vi "2D plot_take linecut_average.vi"() -> ()   [LabVIEW 2016]
uses:
  <vilib>/Analysis/baseanly.llb/Mean (DBL).vi
  <vilib>/Analysis/NI_AALPro.lvlib
  <vilib>/Analysis/NI_AALBase.lvlib
  <vilib>/gmath/NI_Gmath.lvlib
  <userlib>/_OpenG.lib/array/array.llb/Delete Elements from 1D Array (DBL)__ogtk.vi
  <userlib>/_OpenG.lib/array/array.llb/Search 1D Array (DBL)__ogtk.vi
  <vilib>/Analysis/NI_AAL_SigProc.lvlib
panel:
  in  "threshold 2":dbl format="%0.2f"
  in  "width 2":i32=3 min=3
  out "trandconductance 2":cluster{dbl[], dbl[]}[](graph)
  out "Indices of Elements 2":i32[](array[numeric])
  out "Array 3":dbl[](array[numeric])
  out "array w/ subset deleted 2":dbl[](array[numeric]) format="%.2f"
  out "resampled G 3":cluster{dbl[], dbl[]}(graph)
  out "trandconductance":cluster{dbl[], dbl[]}[](graph)
  out "Array":i32[](array[numeric])
  in  "Tab Control":enum32{"Page 1", "Page 2"}(tab)
  in  "Input transconductance":dbl[][](graph)
  in  "Number of cursors":i32[](array[numeric])=[0, 1, 2, 3]
  in  "input cond":dbl[][](graph)
  out "XY Graph":cluster{"xi used":dbl[], "yi":dbl[]}[](graph)
  out "Trans intensity":dbl[][](graph)
  out "G":cluster{dbl[], dbl[]}[](graph)
  out "Cond intensity":dbl[][](graph)
  in  "alpha":dbl=1.0 format="%#_13g"
  out "mean G change":dbl=3.541411002779411 format="%0.2f"
  out "old average G":cluster{dbl[], dbl[]}[](graph)
  out "delta y1":dbl format="%#_6p"
  out "delta y2":dbl format="%#_6p"
  out "resampled G":cluster{dbl[], dbl[]}[](graph)
  out "resampled average G":cluster{dbl[], dbl[]}[](graph)
  in  "max value":dbl
  in  "min value":dbl
  in  "X Step":dbl=0.00025 format="%#_13g"
  in  "pad array T\ninterpolate F":bool
  out "shifted + avg":cluster{dbl[], dbl[]}[](graph)
  # "29.2    .139\n60.4    .129"
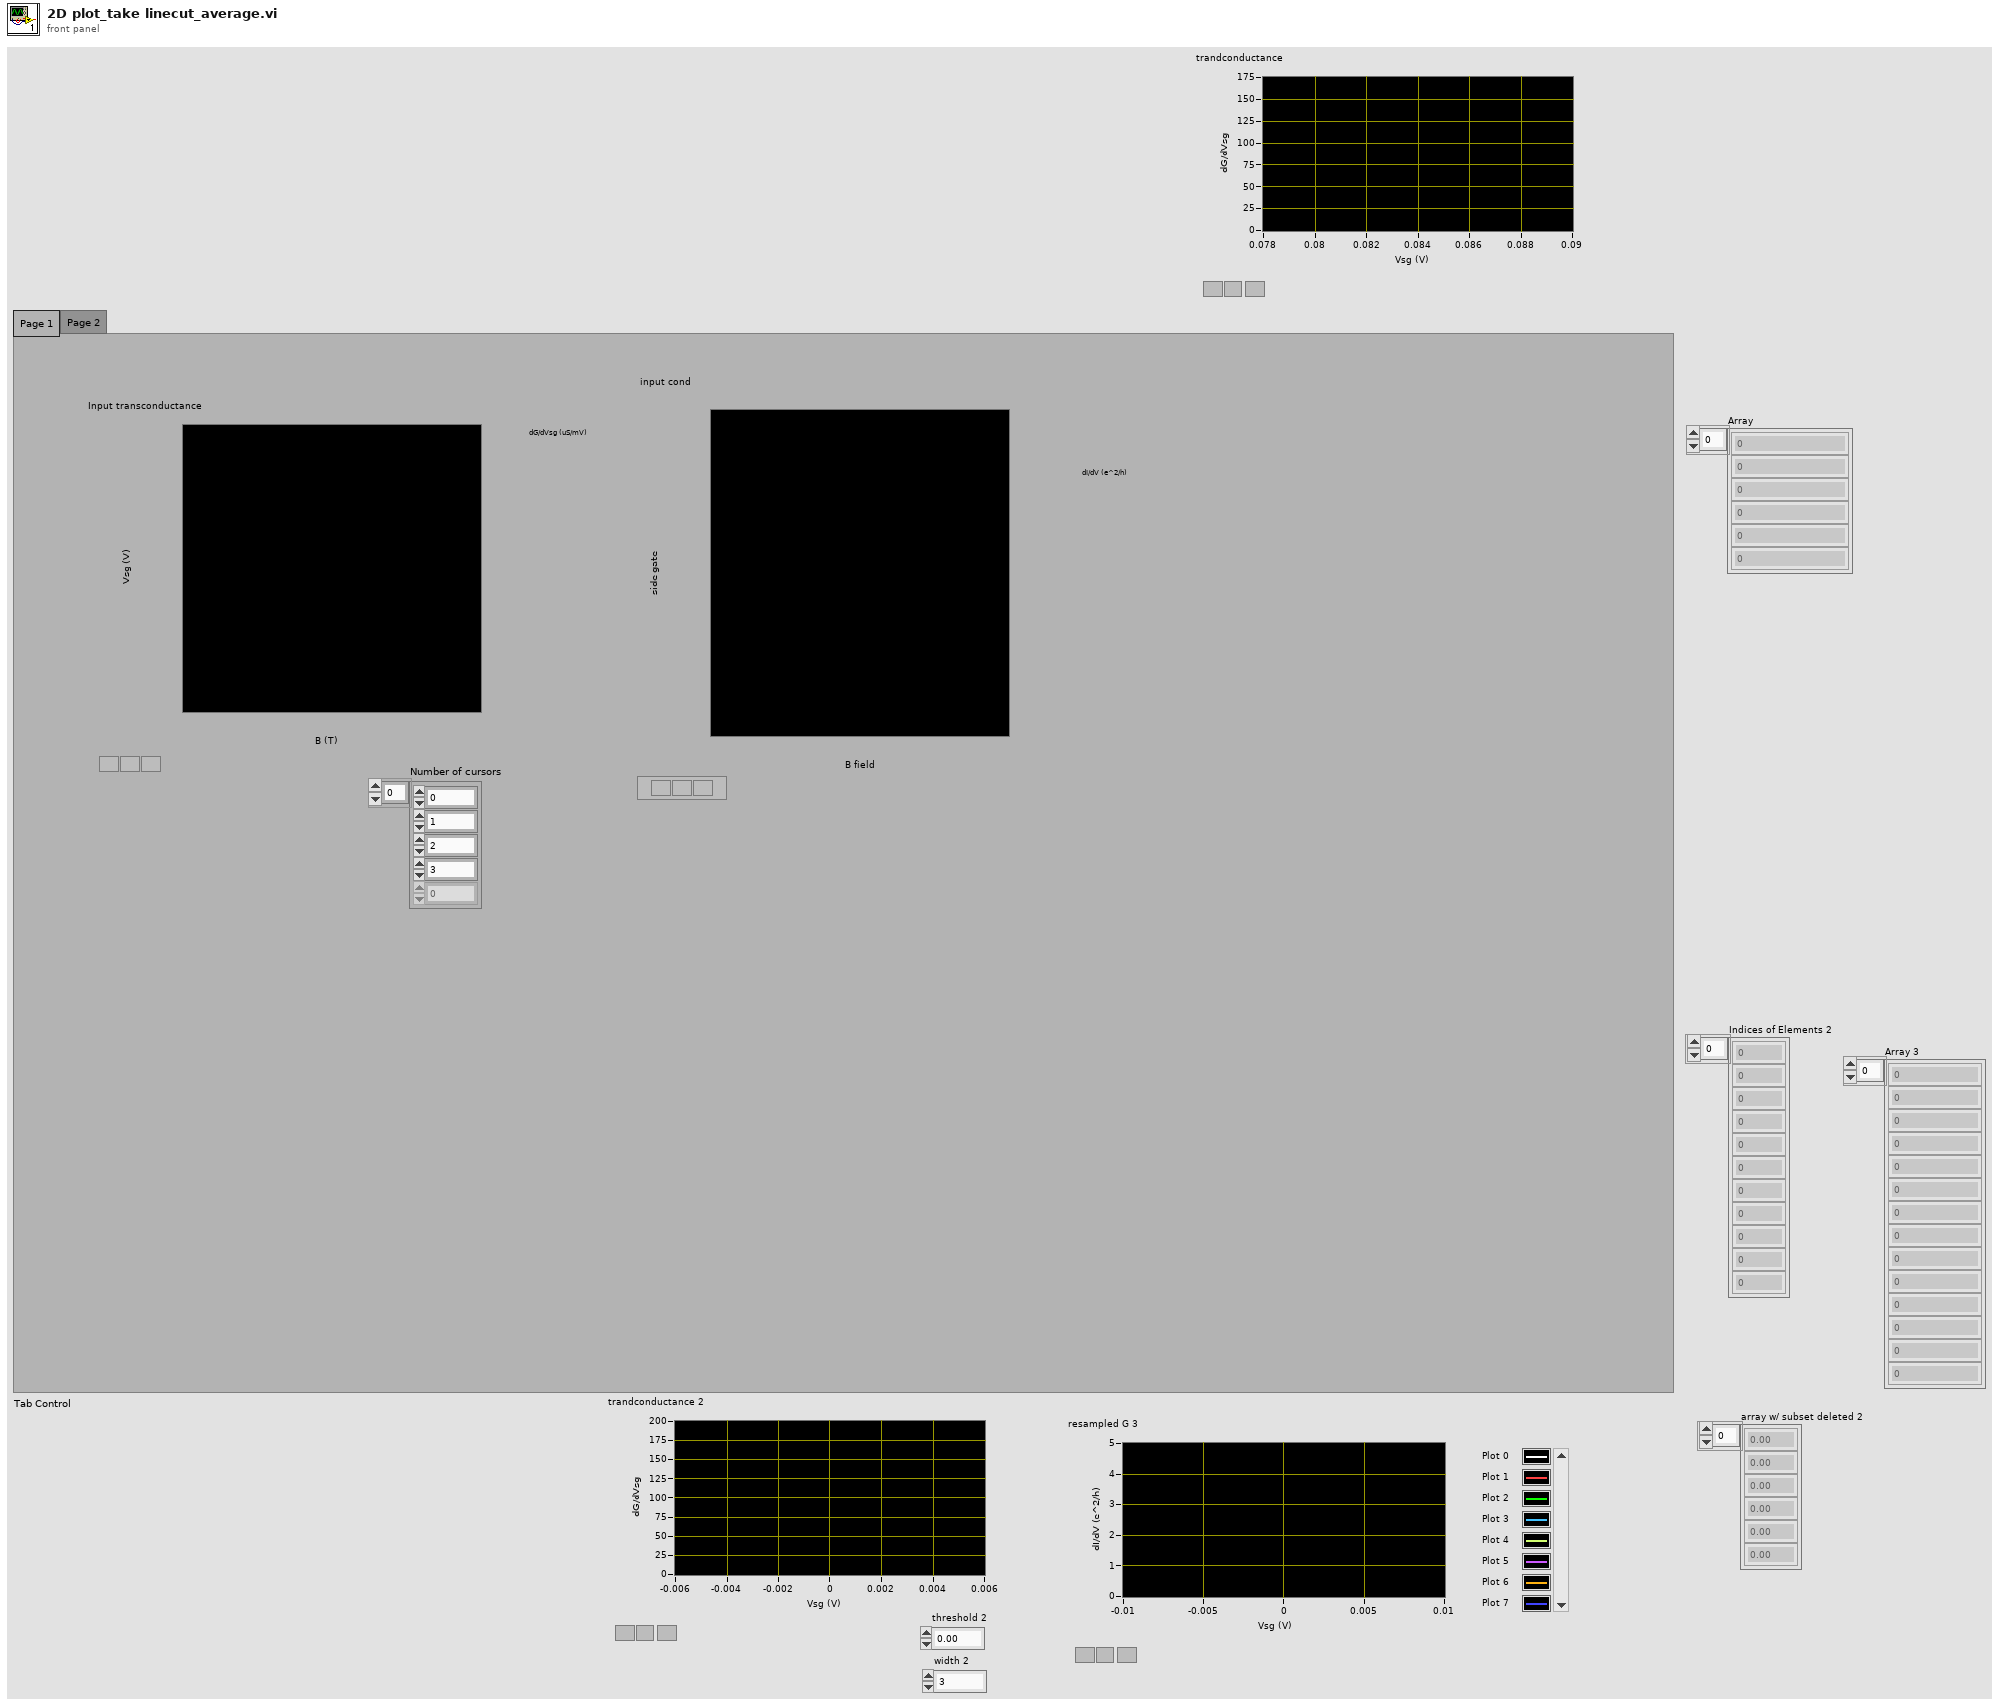
[diagram p1: front panel]
types:
  T1 = typedef "LVOffsetAndMultiplierTypeDef.ctl" = cluster{"Offset":dbl, "Multiplier":dbl}
  T2 = typedef "LVPointDoubleTypeDef.ctl" = cluster{"Cursor X":dbl, "Cursor Y":dbl}
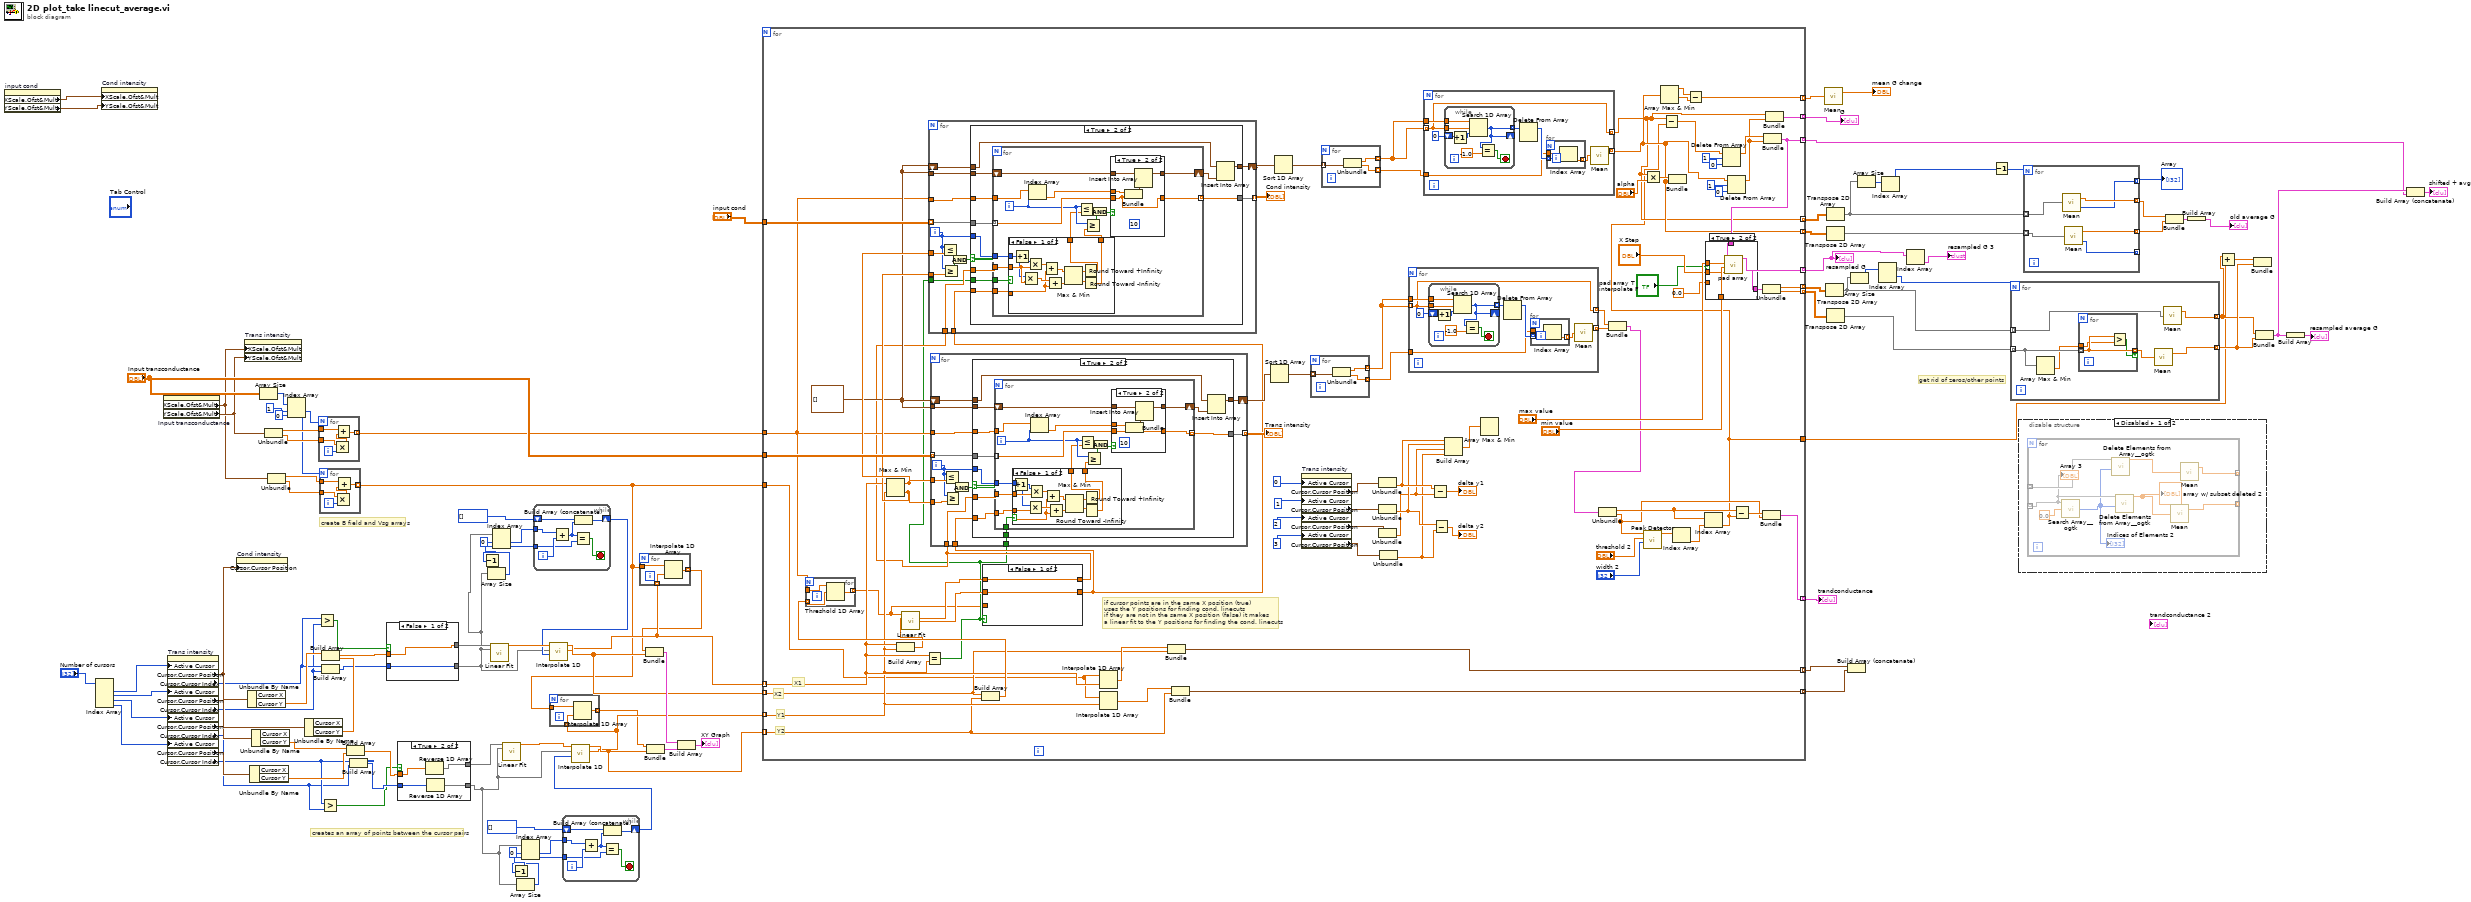
[diagram p0: block diagram]
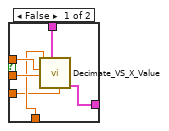
[diagram p3: hidden frame]
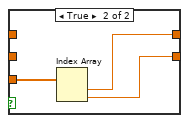
[diagram p4: hidden frame]
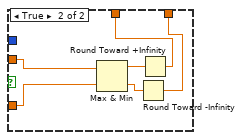
[diagram p6: hidden frame]
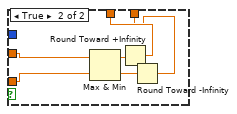
[diagram p9: hidden frame]
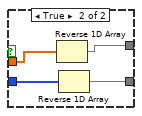
[diagram p12: hidden frame]
diagram:
  # "get rid of zeros/other points"
  # "create B field and Vsg arrays"
  # "creates an array of points between the cursor pairs"
  n1 = property on="input cond" class="IntGraph (strict)"() -> ("XScale.Ofst&Mult"=w89:T1, "YScale.Ofst&Mult"=w88:T1)  [unwired: 2 in, 2 out]
  n2 = Index Array(array="Number of cursors") -> (element #1=w95:i32, element #2=w94:i32, element #3=w87:i32, element #4=w86:i32)  [unwired: 4 in]
  n3 = property on="Cond intensity" class="IntGraph (strict)"("XScale.Ofst&Mult"=w89, "YScale.Ofst&Mult"=w88) -> ()  [unwired: 2 in, 2 out]
  n4 = property on="Input transconductance" class="IntGraph (strict)"() -> ("XScale.Ofst&Mult"=w42:T1, "YScale.Ofst&Mult"=w93:T1)  [unwired: 2 in, 2 out]
  n5 = property on="Trans intensity" class="IntGraph (strict)"("Active Cursor"=w95, "Active Cursor"=w94, "Active Cursor"=w87, "Active Cursor"=w86) -> ("Cursor.Cursor Position"=w90:T2, "Cursor.Cursor Index"=w70:i32, "Cursor.Cursor Position"=w96:T2, "Cursor.Cursor Index"=w69:i32, "Cursor.Cursor Position"=w85:T2, "Cursor.Cursor Index"=w62:i32, "Cursor.Cursor Position"=w84:T2, "Cursor.Cursor Index"=w61:i32)  [unwired: 2 in, 2 out]
  n6 = property on="Cond intensity" class="IntGraph (strict)"("Cursor.Cursor Position"=w90) -> ()  [unwired: 2 in, 2 out]
  n7 = property on="Trans intensity" class="IntGraph (strict)"("XScale.Ofst&Mult"=w42, "YScale.Ofst&Mult"=w93) -> ()  [unwired: 2 in, 2 out]
  n8 = Unbundle By Name(w90) -> ("Cursor Y"=w83:dbl)  [unwired: 1 out]
  n9 = Unbundle By Name(w84) -> ("Cursor Y"=w81:dbl)  [unwired: 1 out]
  n10 = Unbundle By Name(w85) -> ("Cursor Y"=w82:dbl)  [unwired: 1 out]
  n11 = Array Size(array="Input transconductance") -> (size(s)=w101:i32[])
  n12 = Unbundle(w93) -> ("Offset"=w103:dbl, "Multiplier"=w102:dbl)
  n13 = Unbundle(w42) -> ("Offset"=w39:dbl, "Multiplier"=w38:dbl)
  n14 = Index Array(array=w101, index #1=1 ("index"), index #2=0 ("index")) -> (element #1=w98:i32, element #2=w40:i32)
  n15 = Unbundle By Name(w96) -> ("Cursor Y"=w71:dbl)  [unwired: 1 out]
  n16 = for {
    N: w98 -> [_]
    tunnel: w103 -> [w107]
    tunnel: w102 -> [w106]
    tunnel: [w104] -> w91 mode=indexing
    i -> [w108]
    n17 = Multiply(x=w106, y=w108) -> (x*y=w105:dbl)
    n18 = Add(x=w107, y=w105) -> (x+y=w104:dbl)
  }
  n19 = Greater?(x=w70, y=w69) -> (0:w64:bool)
  n20 = for {
    N: w40 -> [_]
    tunnel: w39 -> [w112]
    tunnel: w38 -> [w111]
    tunnel: [w109] -> w35 mode=indexing
    i -> [w113]
    n21 = Multiply(x=w111, y=w113) -> (x*y=w110:dbl)
    n22 = Add(x=w112, y=w110) -> (x+y=w109:dbl)
  }
  n23 = Build Array(w70, w69) -> (w66:i32[])
  n24 = Greater?(x=w62, y=w61) -> (0:w58:bool)
  n25 = Build Array(w83, w71) -> (w68:dbl[])
  n26 = Build Array(w82, w81) -> (w60:dbl[])
  n27 = Build Array(w62, w61) -> (w59:i32[])
  n28 = case shown="False" w64 {
    tunnel: w68 -> [w115 w119]
    tunnel: [w115 w118] -> w67
    tunnel: w66 -> [w114 w117]
    tunnel: [w114 w116] -> w65
    frame False {
    }
    frame True {
      n29 = Reverse 1D Array(array=w119) -> (reversed array=w118:dbl[])
      n30 = Reverse 1D Array(array=w117) -> (reversed array=w116:i32[])
    }
  }
  n31 = case shown="True" w58 {
    tunnel: w60 -> [w121 w125]
    tunnel: [w121 w124] -> w57
    tunnel: w59 -> [w120 w123]
    tunnel: [w120 w122] -> w49
    frame False {
    }
    frame True {
      n32 = Reverse 1D Array(array=w125) -> (reversed array=w124:dbl[])
      n33 = Reverse 1D Array(array=w123) -> (reversed array=w122:i32[])
    }
  }
  n34 = Array Size(array=w65) -> (size(s)=w77:i32)
  n35 = Decrement(x=w77) -> (x-1=w76:i32)
  n36 = call <vilib>:"Linear Fit.vi"("Y"=w67, "X"=w65) -> ("Best Linear Fit"=w79:dbl[])  [unwired: 9 in, 4 out]
  n37 = Index Array(array=w65, index #1=0 ("index"), index #2=w76) -> (element #1=w74:i32, element #2=w73:i32)
  n38 = call <vilib>:"Linear Fit.vi"("Y"=w57, "X"=w49) -> ("Best Linear Fit"=w50:dbl[])  [unwired: 9 in, 4 out]
  n39 = Array Size(array=w49) -> (size(s)=w52:i32)
  n40 = Decrement(x=w52) -> (x-1=w53:i32)
  n41 = Index Array(array=w49, index #1=0 ("index"), index #2=w53) -> (element #1=w55:i32, element #2=w56:i32)
  n42 = while {
    shift-right: [w129] -> w72
    shift-left: i32[] [] -> [w130]
    tunnel: w74 -> [w132]
    tunnel: w73 -> [w126]
    i -> [w131]
    stop <- w128 stop-if-true
    n43 = Add(x=w132, y=w131) -> (x+y=w127:i32)
    n44 = Build Array (concatenate)(w130, w127) -> (w129:i32[])
    n45 = Equal?(x=w127, y=w126) -> (x = y?=w128:bool)
  }
  n46 = call <vilib>:"Interpolate 1D.vi"("xi"=w72, "X"=w65, "Y"=w79) -> ("xi used"=w37:dbl[], "yi"=w46:dbl[])  [unwired: 6 in, 1 out]
  n47 = while {
    shift-right: [w136] -> w48
    shift-left: i32[] [] -> [w137]
    tunnel: w55 -> [w139]
    tunnel: w56 -> [w133]
    i -> [w138]
    stop <- w135 stop-if-true
    n48 = Add(x=w139, y=w138) -> (x+y=w134:i32)
    n49 = Build Array (concatenate)(w137, w134) -> (w136:i32[])
    n50 = Equal?(x=w134, y=w133) -> (x = y?=w135:bool)
  }
  n51 = call <vilib>:"Interpolate 1D.vi"("xi"=w48, "X"=w49, "Y"=w50) -> ("xi used"=w34:dbl[], "yi"=w45:dbl[])  [unwired: 6 in, 1 out]
  n52 = for {
    tunnel: w35 -> [w142]
    tunnel: w34 -> [w141] mode=indexing
    tunnel: [w140] -> w33 mode=indexing
    n53 = Interpolate 1D Array(1:w141, 2:w142) -> (0:w140:dbl)
  }
  n54 = for {
    tunnel: w35 -> [w145]
    tunnel: w37 -> [w144] mode=indexing
    tunnel: [w143] -> w36 mode=indexing
    n55 = Interpolate 1D Array(1:w144, 2:w145) -> (0:w143:dbl)
  }
  n56 = Bundle(w36, "yi"=w46) -> (w63:cluster{dbl[], "yi":dbl[]})  [unwired: 1 in]
  n57 = Bundle(w33, "yi"=w45) -> (w47:cluster{dbl[], "yi":dbl[]})  [unwired: 1 in]
  n58 = Build Array(w63, w47) -> (→"XY Graph":cluster{dbl[], "yi":dbl[]}[])
  n59 = for {
    tunnel: "Input transconductance" -> [w229]
    tunnel: [w150] -> w9 mode=indexing
    tunnel: "input cond" -> [w219]
    tunnel: w91 -> [w206]
    tunnel: w46 -> [w194] mode=indexing
    tunnel: w45 -> [w193] mode=indexing
    tunnel: w37 -> [w200] mode=indexing
    tunnel: w34 -> [w199] mode=indexing
    tunnel: [w208] -> w44 mode=indexing
    tunnel: [w207] -> w43 mode=indexing
    tunnel: w35 -> [w190]
    tunnel: [w201] -> w32 mode=indexing
    tunnel: [w164] -> w7 mode=indexing
    tunnel: [w147] -> w30 mode=indexing
    tunnel: [w160] -> w29 mode=indexing
    tunnel: [w169] -> w11 mode=indexing
    tunnel: [w174] -> w18 mode=indexing
    tunnel: [w173] -> w17 mode=indexing
    tunnel: [w148] -> w1 mode=indexing
    tunnel: [w146] -> w3
    w216 = cluster{dbl, dbl}[] []
    # "if cursor points are in the same X position (true)\nuses the Y positions for finding cond. linecuts\nif they are not in the same X position (false) it makes\na linear fit to the Y positions for finding the cond. linecuts"
    # "X2"
    # "X1"
    # "Y2"
    # "Y1"
    n60 = Max & Min(x=w200, y=w199) -> (max(x,y)=w218:dbl, min(x,y)=w217:dbl)
    n61 = Build Array(w200, w199) -> (w226:dbl[])
    n62 = Equal?(x=w200, y=w199) -> (x = y?=w192:bool)
    n63 = Build Array(w194, w193) -> (w227:dbl[])
    n64 = for {
      tunnel: w206 -> [w428]
      tunnel: w227 -> [w427] mode=indexing
      tunnel: [w426] -> w191 mode=indexing
      n65 = Threshold 1D Array(2:w427, 3:w428) -> (0:w426:dbl)  [unwired: 1 in]
    }
    n66 = call <vilib>:"Linear Fit.vi"("Y"=w191, "X"=w226) -> ("slope"=w198:dbl, "intercept"=w197:dbl)  [unwired: 9 in, 3 out]
    n67 = case shown="False" w192 {
      tunnel: w198 -> [w242 _]
      tunnel: w197 -> [w241 _]
      tunnel: [w242 w244] -> w196
      tunnel: [w241 w243] -> w195
      tunnel: w191 -> [_ w245]
      frame False {
      }
      frame True {
        n68 = Index Array(array=w245) -> (element #1=w244:dbl, element #2=w243:dbl)  [unwired: 2 in]
      }
    }
    n69 = for {
      tunnel: w218 -> [w278]
      tunnel: w217 -> [w277]
      tunnel: w196 -> [w274]
      tunnel: w195 -> [w273]
      tunnel: w219 -> [w276] mode=indexing
      tunnel: [w275] -> w209 mode=indexing
      tunnel: w206 -> [w271]
      shift-right: [w270] -> w215
      shift-left: w216 -> [w269]
      tunnel: w216 -> [w268]
      tunnel: w192 -> [w267]
      i -> [w272]
      n70 = Less Or Equal?(x=w272, y=w278) -> (x <= y?=w280:bool)
      n71 = Greater Or Equal?(x=w272, y=w277) -> (x >= y?=w279:bool)
      n72 = And(x=w280, y=w279) -> (x .and. y?=w281:bool)
      n73 = case shown="True" w281 {
        tunnel: w276 -> [w283 w291]
        tunnel: [w283 w290] -> w275
        tunnel: w274 -> [_ w294]
        tunnel: w272 -> [_ w293]
        tunnel: w273 -> [_ w292]
        tunnel: w271 -> [_ w289]
        tunnel: [w282 w288] -> w270
        tunnel: w269 -> [w282 w287]
        tunnel: w268 -> [_ w286]
        tunnel: w267 -> [_ w284]
        frame False {
        }
        frame True {
          n74 = for {
            tunnel: w294 -> [w308]
            tunnel: w293 -> [w306]
            tunnel: w292 -> [w307]
            tunnel: w291 -> [w310] mode=indexing
            tunnel: [w309] -> w290 mode=indexing
            tunnel: w289 -> [w305]
            shift-right: [w299] -> w285
            shift-left: w286 -> [w298]
            tunnel: w284 -> [w295]
            i -> [w304]
            n75 = case shown="False" w295 {
              tunnel: w308 -> [w321 w328]
              tunnel: w307 -> [w320 w327]
              tunnel: w306 -> [w318 _]
              tunnel: [w312 w324] -> w297
              tunnel: [w311 w323] -> w296
              frame False {
                n76 = Increment(x=w318) -> (x+1=w317:i32)
                n77 = Multiply(x=w318, y=w321) -> (x*y=w322:dbl)
                n78 = Multiply(x=w317, y=w321) -> (x*y=w319:dbl)
                n79 = Add(x=w319, y=w320) -> (x+y=w316:dbl)
                n80 = Add(x=w322, y=w320) -> (x+y=w315:dbl)
                n81 = Max & Min(x=w316, y=w315) -> (max(x,y)=w314:dbl, min(x,y)=w313:dbl)
                n82 = Round Toward +Infinity(x=w314) -> (ceil(x): smallest int >= x=w312:dbl)
                n83 = Round Toward -Infinity(1:w313) -> (0:w311:dbl)
              }
              frame True {
                n84 = Max & Min(x=w328, y=w327) -> (max(x,y)=w326:dbl, min(x,y)=w325:dbl)
                n85 = Round Toward -Infinity(1:w325) -> (0:w323:dbl)
                n86 = Round Toward +Infinity(x=w326) -> (ceil(x): smallest int >= x=w324:dbl)
              }
            }
            n87 = Index Array(array=w305, index=w304) -> (element=w303:dbl)
            n88 = Less Or Equal?(x=w304, y=w297) -> (x <= y?=w302:bool)
            n89 = Greater Or Equal?(x=w304, y=w296) -> (x >= y?=w301:bool)
            n90 = And(x=w302, y=w301) -> (x .and. y?=w300:bool)
            n91 = case shown="True" w300 {
              tunnel: w310 -> [w330 w331]
              tunnel: [w330 w331] -> w309
              tunnel: w303 -> [_ w335]
              tunnel: [w329 w333] -> w299
              tunnel: w298 -> [w329 w332]
              frame False {
              }
              frame True {
                (unwired) 10
                n92 = Bundle(w335, w331) -> (w334:cluster{dbl, dbl})  [unwired: 1 in]
                n93 = Insert Into Array(array=w332, new element=w334) -> (w333:cluster{dbl, dbl}[])  [unwired: 1 in]
              }
            }
          }
          n94 = Insert Into Array(array=w287, new element=w285) -> (w288:cluster{dbl, dbl}[])  [unwired: 1 in]
        }
      }
    }
    "Cond intensity" <- w209
    n95 = for {
      tunnel: w218 -> [w368]
      tunnel: w217 -> [w367]
      tunnel: w196 -> [w364]
      tunnel: w195 -> [w363]
      tunnel: w229 -> [w366] mode=indexing
      tunnel: [w365] -> w228 mode=indexing
      tunnel: w206 -> [w361]
      shift-right: [w360] -> w225
      shift-left: w216 -> [w359]
      tunnel: w216 -> [w358]
      tunnel: w192 -> [w357]
      i -> [w362]
      n96 = Less Or Equal?(x=w362, y=w368) -> (x <= y?=w370:bool)
      n97 = Greater Or Equal?(x=w362, y=w367) -> (x >= y?=w369:bool)
      n98 = And(x=w370, y=w369) -> (x .and. y?=w371:bool)
      n99 = case shown="True" w371 {
        tunnel: w366 -> [w373 w381]
        tunnel: [w373 w380] -> w365
        tunnel: w364 -> [_ w384]
        tunnel: w362 -> [_ w383]
        tunnel: w363 -> [_ w382]
        tunnel: w361 -> [_ w379]
        tunnel: [w372 w378] -> w360
        tunnel: w359 -> [w372 w377]
        tunnel: w358 -> [_ w376]
        tunnel: w357 -> [_ w374]
        frame False {
        }
        frame True {
          n100 = for {
            tunnel: w384 -> [w398]
            tunnel: w383 -> [w396]
            tunnel: w382 -> [w397]
            tunnel: w381 -> [w400] mode=indexing
            tunnel: [w399] -> w380 mode=indexing
            tunnel: w379 -> [w395]
            shift-right: [w389] -> w375
            shift-left: w376 -> [w388]
            tunnel: w374 -> [w385]
            i -> [w394]
            n101 = case shown="False" w385 {
              tunnel: w398 -> [w411 w418]
              tunnel: w397 -> [w410 w417]
              tunnel: w396 -> [w408 _]
              tunnel: [w402 w415] -> w387
              tunnel: [w401 w413] -> w386
              frame False {
                n102 = Increment(x=w408) -> (x+1=w407:i32)
                n103 = Multiply(x=w408, y=w411) -> (x*y=w412:dbl)
                n104 = Multiply(x=w407, y=w411) -> (x*y=w409:dbl)
                n105 = Add(x=w409, y=w410) -> (x+y=w406:dbl)
                n106 = Add(x=w412, y=w410) -> (x+y=w405:dbl)
                n107 = Max & Min(x=w406, y=w405) -> (max(x,y)=w404:dbl, min(x,y)=w403:dbl)
                n108 = Round Toward +Infinity(x=w404) -> (ceil(x): smallest int >= x=w402:dbl)
                n109 = Round Toward -Infinity(1:w403) -> (0:w401:dbl)
              }
              frame True {
                n110 = Max & Min(x=w418, y=w417) -> (max(x,y)=w416:dbl, min(x,y)=w414:dbl)
                n111 = Round Toward +Infinity(x=w416) -> (ceil(x): smallest int >= x=w415:dbl)
                n112 = Round Toward -Infinity(1:w414) -> (0:w413:dbl)
              }
            }
            n113 = Index Array(array=w395, index=w394) -> (element=w393:dbl)
            n114 = Less Or Equal?(x=w394, y=w387) -> (x <= y?=w392:bool)
            n115 = Greater Or Equal?(x=w394, y=w386) -> (x >= y?=w391:bool)
            n116 = And(x=w392, y=w391) -> (x .and. y?=w390:bool)
            n117 = case shown="True" w390 {
              tunnel: w400 -> [w420 w421]
              tunnel: [w420 w421] -> w399
              tunnel: w393 -> [_ w425]
              tunnel: [w419 w423] -> w389
              tunnel: w388 -> [w419 w422]
              frame False {
              }
              frame True {
                (unwired) 10
                n118 = Bundle(w425, w421) -> (w424:cluster{dbl, dbl})  [unwired: 1 in]
                n119 = Insert Into Array(array=w422, new element=w424) -> (w423:cluster{dbl, dbl}[])  [unwired: 1 in]
              }
            }
          }
          n120 = Insert Into Array(array=w377, new element=w375) -> (w378:cluster{dbl, dbl}[])  [unwired: 1 in]
        }
      }
    }
    "Trans intensity" <- w228
    n121 = Interpolate 1D Array(1:w200, 2:w190) -> (0:w204:dbl)
    n122 = Interpolate 1D Array(1:w199, 2:w190) -> (0:w205:dbl)
    n123 = Bundle(w204, "Numeric"=w194) -> (w208:cluster{dbl, "Numeric":dbl})  [unwired: 1 in]
    n124 = Bundle(w205, "Numeric"=w193) -> (w207:cluster{dbl, "Numeric":dbl})  [unwired: 1 in]
    n125 = Sort 1D Array(array=w225) -> (sorted array=w224:cluster{dbl, dbl}[])
    n126 = Sort 1D Array(array=w215) -> (sorted array=w214:cluster{dbl, dbl}[])
    n127 = property on="Trans intensity" class="IntGraph (strict)"("Active Cursor"=0, "Active Cursor"=1, "Active Cursor"=2, "Active Cursor"=3) -> ("Cursor.Cursor Position"=w185:T2, "Cursor.Cursor Position"=w184:T2, "Cursor.Cursor Position"=w183:T2, "Cursor.Cursor Position"=w182:T2)  [unwired: 2 in, 2 out]
    n128 = for {
      tunnel: w224 -> [w356] mode=indexing
      tunnel: [w355] -> w223 mode=indexing
      tunnel: [w354] -> w222 mode=indexing
      n129 = Unbundle(w356) -> (w355:dbl, w354:dbl)
    }
    n130 = for {
      tunnel: w214 -> [w266] mode=indexing
      tunnel: [w265] -> w213 mode=indexing
      tunnel: [w264] -> w212 mode=indexing
      n131 = Unbundle(w266) -> (w265:dbl, w264:dbl)
    }
    n132 = Unbundle(w185) -> ("Cursor Y"=w179:dbl)  [unwired: 1 out]
    n133 = Unbundle(w184) -> ("Cursor Y"=w178:dbl)  [unwired: 1 out]
    n134 = Unbundle(w183) -> ("Cursor Y"=w177:dbl)  [unwired: 1 out]
    n135 = Unbundle(w182) -> ("Cursor Y"=w176:dbl)  [unwired: 1 out]
    n136 = for {
      tunnel: w223 -> [w341]
      tunnel: w223 -> [w336] mode=indexing
      tunnel: w222 -> [w338]
      tunnel: [w337] -> w221 mode=indexing
      tunnel: [w336] -> w220 mode=indexing
      n137 = while {
        tunnel: w341 -> [w353]
        tunnel: w336 -> [w352]
        shift-right: [w347] -> _
        shift-left: 0 ("index of element") -> [w349]
        tunnel: [w347] -> w342 mode=indexing
        stop <- w350 stop-if-true
        n138 = Increment(x=w349) -> (x+1=w348:i32)
        n139 = Search 1D Array(1D array=w353, element=w352, start index (0)=w348) -> (index of element=w347:i32)
        n140 = Equal?(x=w347, y=-1.0) -> (x = y?=w350:bool)
      }
      n141 = Delete From Array(array=w342) -> (array with subset deleted=w340:i32[])  [unwired: 2 in, 1 out]
      n142 = for {
        tunnel: w338 -> [w346]
        tunnel: w340 -> [w345] mode=indexing
        tunnel: [w344] -> w339 mode=indexing
        n143 = Index Array(array=w346, index=w345) -> (element=w344:dbl)
      }
      n144 = call-poly <vilib>:"Mean.vi"("X"=w339) -> ("mean"=w337:dbl)  [unwired: 1 out]
    }
    n145 = for {
      tunnel: w213 -> [w251]
      tunnel: w213 -> [w246] mode=indexing
      tunnel: w212 -> [w248]
      tunnel: [w247] -> w160 mode=indexing
      tunnel: [w246] -> w147 mode=indexing
      n146 = while {
        tunnel: w251 -> [w263]
        tunnel: w246 -> [w262]
        shift-right: [w257] -> _
        shift-left: 0 ("index of element") -> [w259]
        tunnel: [w257] -> w252 mode=indexing
        stop <- w260 stop-if-true
        n147 = Increment(x=w259) -> (x+1=w258:i32)
        n148 = Search 1D Array(1D array=w263, element=w262, start index (0)=w258) -> (index of element=w257:i32)
        n149 = Equal?(x=w257, y=-1.0) -> (x = y?=w260:bool)
      }
      n150 = Delete From Array(array=w252) -> (array with subset deleted=w250:i32[])  [unwired: 2 in, 1 out]
      n151 = for {
        tunnel: w248 -> [w256]
        tunnel: w250 -> [w255] mode=indexing
        tunnel: [w254] -> w249 mode=indexing
        n152 = Index Array(array=w256, index=w255) -> (element=w254:dbl)
      }
      n153 = call-poly <vilib>:"Mean.vi"("X"=w249) -> ("mean"=w247:dbl)  [unwired: 1 out]
    }
    n154 = Subtract(x=w179, y=w177) -> (x-y=→"delta y1":dbl)
    n155 = Subtract(x=w178, y=w176) -> (x-y=→"delta y2":dbl)
    n156 = Build Array(w179, w178, w177, w176) -> (w175:dbl[])
    n157 = Array Max & Min(array=w175) -> ()  [unwired: 4 out]
    n158 = Bundle(w220, w221) -> (w152:cluster{dbl[], dbl[]})  [unwired: 1 in]
    n159 = Unbundle(w152) -> (w155:dbl[], w153:dbl[])
    n160 = call <vilib>:"Peak Detector.vi"("width"="width 2", "threshold"="threshold 2", "X"=w153) -> ("Locations"=w157:dbl[])  [unwired: 4 in, 4 out]
    n161 = Multiply(x=w147, y="alpha") -> (x*y=w210:dbl[])
    n162 = Array Max & Min(array=w160) -> (max value=w203:dbl, min value=w202:dbl)  [unwired: 2 out]
    n163 = Bundle(w210, w160) -> ()  [unwired: 1 in, 1 out]
    n164 = Index Array(array=w157) -> (element=w156:dbl)  [unwired: 1 in]
    n165 = Subtract(x=w203, y=w202) -> (x-y=w201:dbl)
    n166 = Index Array(array=w155, index=w156) -> (element=w146:dbl)
    n167 = Subtract(x=w147, y=w146) -> (x-y=w151:dbl[])
    n168 = Delete From Array(array=w151, length=1, index=0) -> (array with subset deleted=w163:dbl[])  [unwired: 1 out]
    n169 = Delete From Array(array=w160, length=1, index=0) -> (array with subset deleted=w149:dbl[])  [unwired: 1 out]
    n170 = Subtract(x=w155, y=w146) -> (x-y=w154:dbl[])
    n171 = Bundle(w154, w153) -> (w150:cluster{dbl[], dbl[]})  [unwired: 1 in]
    n172 = Bundle(w163, w149) -> (w164:cluster{dbl[], dbl[]})  [unwired: 1 in]
    n173 = case shown="True" "pad array T\ninterpolate F" {
      tunnel: w164 -> [w235 w240]
      tunnel: "max value" -> [w232 w239]
      tunnel: "min value" -> [w231 w238]
      tunnel: "X Step" -> [w233 w237]
      tunnel: [w234 w236] -> w169
      tunnel: 0.0 ("fake point value") -> [w230 _]
      frame False {
        n174 = call <userlib>:"Decimate_VS_X_Value.vi"("fake point value"=w230, "XY Graph kind 1"=w235, "X Step"=w233, "X High"=w232, "X Low"=w231) -> ("Interpolated"=w234:cluster{dbl[], dbl[]})  [unwired: 5 in, 1 out]
      }
      frame True {
        n175 = call "pad array.vi"("X Step"=w237, "min value"=w238, "max value"=w239, "G 2"=w240) -> ("G 3"=w236:cluster{dbl[], dbl[]})  [unwired: 7 in]
      }
    }
    n176 = Unbundle(w169) -> (w174:dbl[], w173:dbl[])
    n177 = Bundle(w147, w149) -> (w148:cluster{dbl[], dbl[]})  [unwired: 1 in]
  }
  "trandconductance" <- w9
  "G" <- w1
  "resampled G" <- w11
  n178 = call-poly <vilib>:"Mean.vi"("X"=w32) -> ("mean"=→"mean G change":dbl)  [unwired: 1 out]
  n179 = Transpose 2D Array(2D array=w18) -> (transposed array=w14:dbl[][])
  n180 = Transpose 2D Array(2D array=w30) -> (transposed array=w24:dbl[][])
  n181 = Transpose 2D Array(2D array=w29) -> (transposed array=w28:dbl[][])
  n182 = Transpose 2D Array(2D array=w17) -> (transposed array=w16:dbl[][])
  n183 = Build Array (concatenate)(w44, w43) -> ()  [unwired: 1 out]
  n184 = Array Size(array=w14) -> (size(s)=w15:i32[])
  n185 = Array Size(array=w24) -> (size(s)=w23:i32[])
  n186 = Index Array(array=w15) -> (element #1=w12:i32)  [unwired: 2 in, 1 out]
  n187 = Index Array(array=w23) -> (element=w22:i32)  [unwired: 1 in]
  n188 = Index Array(array=w11) -> (element=→"resampled G 3":cluster{dbl[], dbl[]})  [unwired: 1 in]
  n189 = Decrement(x=w22) -> (x-1=w21:i32)
  n190 = for {
    N: w12 -> [_]
    tunnel: w14 -> [w429] mode=indexing
    tunnel: w16 -> [w432] mode=indexing
    tunnel: [w434] -> w5 mode=indexing
    tunnel: [w433] -> w4 mode=indexing
    n191 = Array Max & Min(array=w432) -> (min value=w431:dbl)  [unwired: 3 out]
    n192 = for {
      tunnel: w432 -> [w437] mode=indexing
      tunnel: [w437] -> w430 mode=indexing if=w436
      tunnel: w431 -> [w435]
      n193 = Greater?(x=w437, y=w435) -> (0:w436:bool)
    }
    n194 = call-poly <vilib>:"Mean.vi"("X"=w430) -> ("mean"=w434:dbl)  [unwired: 1 out]
    n195 = call-poly <vilib>:"Mean.vi"("X"=w429) -> ("mean"=w433:dbl)  [unwired: 1 out]
  }
  n196 = disable-structure shown="Disabled" {
    frame Disabled {
      n197 = for {
        tunnel: _ -> [w443] mode=indexing
        tunnel: _ -> [w440] mode=indexing
        tunnel: [w445] -> _ mode=indexing
        tunnel: [w444] -> _ mode=indexing
        n198 = call-poly <userlib>:"Search Array__ogtk.vi"("Array"=w440, "Element Data"=0.0 ("element")) -> ("Indices of Elements"=w439:i32[])  [unwired: 7 in]
        "Indices of Elements 2" <- w439
        n199 = call-poly <userlib>:"Delete Elements from Array__ogtk.vi"("indices"=w439, "array"=w443) -> ("array w/ subset deleted"=w442:dbl[])  [unwired: 8 in, 1 out]
        n200 = call-poly <userlib>:"Delete Elements from Array__ogtk.vi"("indices"=w439, "array"=w440) -> ("array w/ subset deleted"=w438:dbl[])  [unwired: 8 in, 1 out]
        "array w/ subset deleted 2" <- w438
        n201 = call-poly <vilib>:"Mean.vi"("X"=w438) -> ("mean"=w445:dbl)  [unwired: 1 out]
        n202 = call-poly <vilib>:"Mean.vi"("X"=w442) -> ("mean"=w444:dbl)  [unwired: 1 out]
        "Array 3" <- w440
      }
    }
    frame Enabled {
    }
  }
  n203 = for {
    N: w21 -> [_]
    tunnel: w24 -> [w451] mode=indexing
    tunnel: w28 -> [w450] mode=indexing
    tunnel: [w449] -> w26 mode=indexing
    tunnel: [w448] -> w27 mode=indexing
    tunnel: [w447] -> w19 mode=indexing
    tunnel: [w446] -> _ mode=indexing
    n204 = call-poly <vilib>:"Mean.vi"("X"=w451) -> ("mean"=w448:dbl, "error"=w447:i32)
    n205 = call-poly <vilib>:"Mean.vi"("X"=w450) -> ("mean"=w449:dbl, "error"=w446:i32)
  }
  "Array" <- w19
  n206 = Bundle(w27, w26) -> (w25:cluster{dbl[], dbl[]})  [unwired: 1 in]
  n207 = Build Array(w25) -> (→"old average G":cluster{dbl[], dbl[]}[])
  n208 = Add(x=w4, y=w3) -> (x+y=w2:dbl[])
  n209 = Bundle(w2, w5) -> ()  [unwired: 1 in, 1 out]
  n210 = Bundle(w4, w5) -> (w8:cluster{dbl[], dbl[]})  [unwired: 1 in]
  n211 = Build Array(w8) -> (→"resampled average G":cluster{dbl[], dbl[]}[])
  n212 = Build Array (concatenate)(w8, w7) -> (→"shifted + avg":cluster{dbl[], dbl[]}[])
